vi "Check if Icon Specified.vi"(1 "Icon Text":T1={"Line 1 text"="Bus", "Line 2 text"="Dev", "Line 3 text"="Ch", "Line 4 text"=""}) -> (0 "No Icon Specified":bool)   [LabVIEW 2014]
doc: "Checks if all items in Icon Text cluster are empty. If all are empty, no icon text has been specified."
uses:
  <vilib>/LabVIEW Icon API/API_Text.ctl
  <vilib>/LabVIEW Icon API/LabVIEW Icon API.lvlib
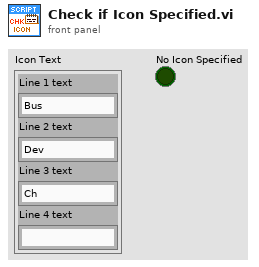
[diagram p1: front panel]
types:
  T1 = typedef "LabVIEW Icon API.lvlib/API_Text.ctl" = cluster{"Line 1 text":string, "Line 2 text":string, "Line 3 text":string, "Line 4 text":string}
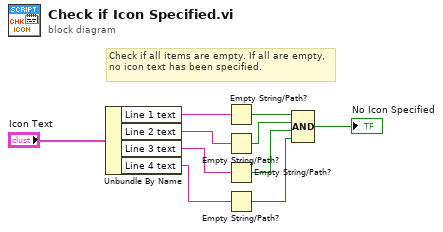
[diagram p0: block diagram]
diagram:
  # "Check if all items are empty. If all are empty, no icon text has been specified."
  n1 = Unbundle By Name("Icon Text") -> ("Line 1 text"=w9:string, "Line 2 text"=w8:string, "Line 3 text"=w7:string, "Line 4 text"=w6:string)
  n2 = Empty String/Path?(string/path=w9) -> (empty?=w5:bool)
  n3 = Empty String/Path?(string/path=w8) -> (empty?=w4:bool)
  n4 = Empty String/Path?(string/path=w7) -> (empty?=w3:bool)
  n5 = Empty String/Path?(string/path=w6) -> (empty?=w2:bool)
  n6 = Compound Arithmetic op=AND(w5, w4, w3, w2) -> (→"No Icon Specified":bool)
